vi "BuildTree.vi"(8 "error in (no error)":errorcluster, 9 "Wired-in Class Refnum":refnum<vi>, 10 "Method Refnum":refnum<vi>, 11 "Tree Refnum":refnum<vi>) -> (0 "error out":errorcluster, 1 "Class To VI Path Map":T1[](array[typedef]), 2 "Nearest Implementation":refnum<vi>, 3 "Tree Refnum out":refnum<vi>, 4 "All Classes":refnum<vi>[](array[refnum]))   [LabVIEW 2017, in "DynamicDispatchImplementationWalker.lvlib"]
uses:
  DynamicDispatchImplementationWalker.lvlib
  TreeSerializer/KeyValuePair.ctl
  TreeItem.ctl
  TreeSerializer/TreeSerializer.lvlib
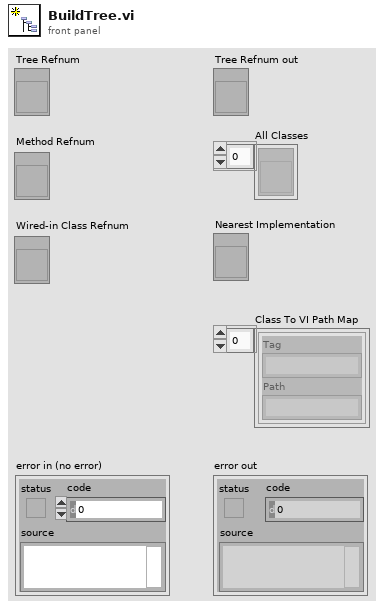
[diagram p1: front panel]
types:
  T1 = typedef "TreeSerializer.lvlib/KeyValuePair.ctl" = cluster{"Tag":string, "Path":string}
  T2 = typedef "DynamicDispatchImplementationWalker.lvlib/TreeItem.ctl" = cluster{"ClassRef":refnum<vi>, "Implementor?":bool, "Parent ItemID":string, "Path":string}
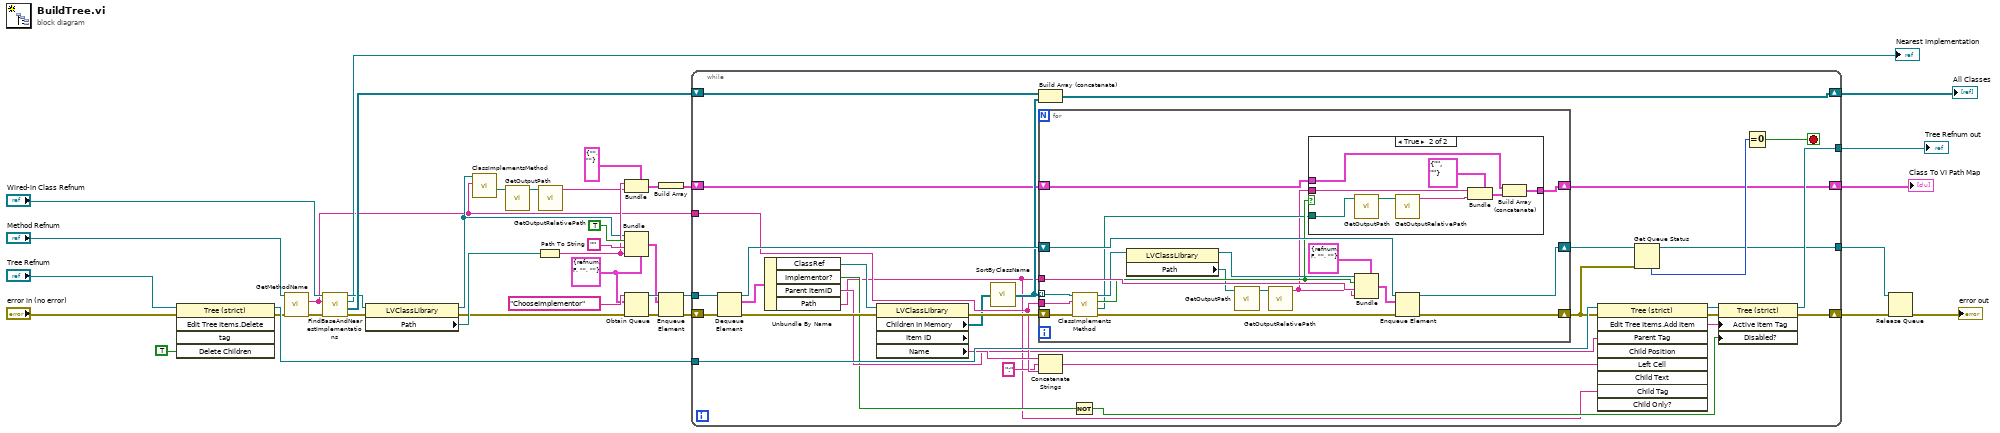
[diagram p0: block diagram]
diagram:
  w30 = T2 {"ClassRef"=refnum, "Implementor?"=FALSE, "Parent ItemID"="", "Path"=""} ("Cluster")
  n1 = invoke class="Tree (strict)" method="Edit Tree Items.Delete"(reference="Tree Refnum", error in="error in (no error)", "Delete Children"=TRUE ("Delete Children?")) -> (reference out=w28:refnum<vi>, error out=w21:errorcluster)  [unwired: 2 in, 3 out]
  n2 = call "GetMethodName.vi"("error in (no error)"=w21, "VI Reference"="Method Refnum") -> ("error out"=w23:errorcluster, "Method Name"=w6:string)  [unwired: 7 in, 1 out]
  n3 = call "FindBaseAndNearestImplementations.vi"("error in (no error)"=w23, "Method Name"=w6, "LVClassLibrary in"="Wired-in Class Refnum") -> ("error out"=w11:errorcluster, "Opened Refs"=w19:refnum<vi>[], "Nearest Implementation"=→"Nearest Implementation":refnum<vi>, "Base Implementation"=w13:refnum<vi>)  [unwired: 5 in]
  n4 = property class="LVClassLibrary"(reference=w13, error in=w11) -> (reference out=w7:refnum<vi>, error out=w10:errorcluster, "Path"=w16:path)
  n5 = call "ClassImplementsMethod.vi"("Method Name"=w6, "Class Refnum"=w7) -> ("Path"=w5:path)  [unwired: 6 in, 3 out]
  n6 = call "GetOutputPath.vi"("Path"=w5) -> ("Output Path"=w4:path)  [unwired: 10 in]
  n7 = Path To String(path=w16) -> (string=w8:string)
  n8 = call "GetOutputRelativePath.vi"("Path"=w4) -> ("Output relative path"=w3:string)  [unwired: 9 in, 1 out]
  n9 = Bundle(cluster=T1 {"Tag"="", "Path"=""} ("Cluster"), "Tag"=w8, "Path"=w3) -> (w2:T1)
  n10 = Bundle(cluster=w30, "ClassRef"=w7, "Implementor?"=TRUE, "Parent ItemID"="", "Path"=w8) -> (w34:T2)
  n11 = Obtain Queue(name (unnamed)="ChooseImplementor", element data type=w30, error in (no error)=w10) -> (queue out=w36:refnum<queue>, error out=w35:errorcluster)  [unwired: 2 in, 1 out]
  n12 = Build Array(w2) -> (w1:T1[])
  n13 = Enqueue Element(queue=w36, element=w34, error in (no error)=w35) -> (queue out=w33:refnum<queue>, error out=w32:errorcluster)  [unwired: 1 in, 1 out]
  n14 = while {
    tunnel: w33 -> [w70]
    shift-right: [w49] -> w18
    shift-left: w32 -> [w69]
    tunnel: w6 -> [w58]
    tunnel: w28 -> [w60]
    tunnel: [w48] -> w26
    tunnel: [w47] -> w22
    shift-right: [w44] -> w17
    shift-left: w19 -> [w45]
    shift-right: [w40] -> w14
    shift-left: w1 -> [w41]
    stop <- w68 stop-if-true
    n15 = Dequeue Element(queue=w70, error in (no error)=w69) -> (queue out=w63:refnum<queue>, element=w66:T2, error out=w64:errorcluster)  [unwired: 1 in, 1 out]
    n16 = Unbundle By Name(w66) -> ("ClassRef"=w65:refnum<vi>, "Implementor?"=w50:bool, "Parent ItemID"=w56:string, "Path"=w39:string)
    n17 = property class="LVClassLibrary" props=["Children In Memory", "Item ID", "Name"](reference=w65, error in=w64) -> (error out=w62:errorcluster, "Children In Memory"=w43:refnum<vi>[], "Name"=w59:string)  [unwired: 2 out]
    n18 = call "SortByClassName.vi"("Children In Memory"=w43) -> ("Sorted Array"=w42:refnum<vi>[])
    n19 = Build Array (concatenate)(w45, w42) -> (w44:refnum<vi>[])
    n20 = for {
      tunnel: w42 -> [w86] mode=indexing
      shift-right: [w81] -> w46
      shift-left: w62 -> [w85]
      tunnel: w39 -> [w87]
      tunnel: w58 -> [w84]
      shift-right: [w83] -> w61
      shift-left: w63 -> [w89]
      shift-right: [w75] -> w40
      shift-left: w41 -> [w76]
      n21 = call "ClassImplementsMethod.vi"("error in (no error)"=w85, "Method Name"=w84, "Class Refnum"=w86) -> ("error out"=w82:errorcluster, "Path"=w77:path, "Implements method?"=w78:bool, "Class Refnum out"=w80:refnum<vi>)  [unwired: 5 in]
      n22 = property class="LVClassLibrary"(reference=w80) -> (reference out=w79:refnum<vi>, "Path"=w72:path)  [unwired: 1 in, 1 out]
      n23 = call "GetOutputPath.vi"("Path"=w72) -> ("Output Path"=w73:path)  [unwired: 10 in]
      n24 = call "GetOutputRelativePath.vi"("Path"=w73) -> ("Output relative path"=w71:string)  [unwired: 9 in, 1 out]
      n25 = case shown="True" w78 {
        tunnel: w71 -> [_ w96]
        tunnel: w77 -> [_ w93]
        tunnel: w76 -> [w90 w98]
        tunnel: [w90 w94] -> w75
        frame False {
        }
        frame True {
          n26 = call "GetOutputPath.vi"("Path"=w93) -> ("Output Path"=w91:path)  [unwired: 10 in]
          n27 = call "GetOutputRelativePath.vi"("Path"=w91) -> ("Output relative path"=w92:string)  [unwired: 9 in, 1 out]
          n28 = Bundle(cluster=T1 {"Tag"="", "Path"=""} ("Cluster"), "Tag"=w96, "Path"=w92) -> (w95:T1)
          n29 = Build Array (concatenate)(w98, w95) -> (w94:T1[])
        }
      }
      n30 = Bundle(cluster=T2 {"ClassRef"=refnum, "Implementor?"=FALSE, "Parent ItemID"="", "Path"=""} ("Cluster"), "ClassRef"=w79, "Implementor?"=w78, "Parent ItemID"=w87, "Path"=w71) -> (w88:T2)
      n31 = Enqueue Element(queue=w89, element=w88, error in (no error)=w82) -> (queue out=w83:refnum<queue>, error out=w81:errorcluster)  [unwired: 1 in, 1 out]
    }
    n32 = Concatenate Strings(w59, ":" ("element"), w58) -> (w55:string)
    n33 = Not(x=w50) -> (.not. x?=w51:bool)
    n34 = invoke class="Tree (strict)" method="Edit Tree Items.Add Item"(reference=w60, error in=w46, "Parent Tag"=w56, "Left Cell"=w55, "Child Tag"=w39) -> (reference out=w54:refnum<vi>, error out=w53:errorcluster, "Edit Tree Items:Add Item"=w52:string)  [unwired: 4 in, 6 out]
    n35 = Get Queue Status(queue=w61, error in (no error)=w46) -> (queue out=w47:refnum<queue>, # elements in queue=w67:i32)  [unwired: 1 in, 6 out]
    n36 = property class="Tree (strict)"(reference=w54, error in=w53, "Active Item Tag"=w52, "Disabled?"=w51) -> (reference out=w48:refnum<vi>, error out=w49:errorcluster)
    n37 = Equal To 0?(x=w67) -> (x = 0?=w68:bool)
  }
  "Tree Refnum out" <- w26
  "All Classes" <- w17
  "Class To VI Path Map" <- w14
  n38 = Release Queue(queue=w22, error in (no error)=w18) -> (error out=→"error out":errorcluster)  [unwired: 1 in, 2 out]
